vi "ECG AF SPI Input.vi"() -> ()   [LabVIEW 2017]
uses:
  <vilib>/Platform/TimedLoop/XDataNode/wakeup.ctl
  <vilib>/Platform/TimedLoop/XDataNode/XDNodeRunTimeDep.lvlib
  <vilib>/Platform/TimedLoop/XDataNode/nitl_modes.ctl
  <vilib>/Platform/TimedLoop/XDataNode/timing_clust.ctl
  <vilib>/Platform/TimedLoop/XDataNode/XDataNode.xnode
  <vilib>/eio/EIONode/EIONode.xnode
  <vilib>/rvi/eio/common/nirviEmuTemplateMethod_errors.vi
  <vilib>/rvi/Analysis/measure/butterworth/XNode/niFpgaButterworthFilter.xnode
  <vilib>/rvi/Analysis/measure/LMRsmpl/XNode/niFPGA Rational Resampler.xnode
  <vilib>/rvi/LocalResourceManager/LocalResourceManager.xnode
  <vilib>/rvi/DataTransferAndStorage/Container/XNode/niFpgaContainer.xnode
  <vilib>/rvi/FIFO/Fifo_Resource/niFpgaFifoEmulationRefIn.vi
  <vilib>/eio/EIOMethodNode/EIOMethodNode.xnode
  <vilib>/rvi/Analysis/common/codeGenErrors/XNode/niFpgaXNodeCodeGenErrorHandle.vi
  ECG Data.ctl
  Gradient Data.ctl
  All Data.ctl
  IBP Data.ctl
  <vilib>/rvi/DataTransferAndStorage/Container/Common/niFpgaContainerGetUniqueNameForEmu.vi
  <vilib>/rvi/DataTransferAndStorage/Container/Common/niFpgaContainerSetEmuInfo.vi
  <vilib>/rvi/eio/common/nirviEmuReportErrorAndStop.vi
  Trigger Params.ctl
  Channel Enum.ctl
panel:
  in  "IBP Filter":bool
  in  "IBP Offset":fxp<+/-,16,16>
  in  "IBP Scale":fxp<+/-,16,5>=1.0
  in  "Offset":cluster{"X":i16, "Y":i16, "Z":i16}
  in  "Beta IBP":fxp<+/-,32,-16>
  out "IPB1 In":i16
  out "IBP2 In":i16
  out "IPB1 Out":i16
  out "IBP2 Out":i16
  in  "ECG Scale":i16=1 min=1 max=100 step=1
  out "LL Out":i16
  out "LA Out":i16
  out "RA Out":i16
  out "LL In":i16
  out "LA In":i16
  out "RA In":i16
  in  "HPF":bool
  in  "Trigger":T1
  out "IBP Data":T3
  out "ECG Data":T4
  in  "Stop":bool
  in  "Reset":bool
  out "Send":bool
  out "WeightSum":fxp<+/-,33,19> format="%.20g"
  out "BetaProduct":fxp<+/-,32,-1> format="%.33g"
  out "Loop Time":u32
  in  "Filter Size":i16
  out "I In":i16
  out "II In":i16
  out "III In":i16
  out "aVR In":i16
  out "aVL In":i16
  out "aVF In":i16
  out "V1 In":i16
  out "V2 In":i16
  out "V3 In":i16
  out "V4 In":i16
  out "V5 In":i16
  out "V6 In":i16
  out "V4 Out":i16
  out "V5 Out":i16
  out "V6 Out":i16
  out "IBP3":i16
  out "IBP2":i16
  out "IBP1":i16
  in  "Start":bool
  in  "ECG Filter":bool=TRUE
  in  "Beta ECG":fxp<+/-,32,-16>
  out "V3 Out":i16
  out "V2 Out":i16
  out "V1 Out":i16
  out "aVF Out":i16
  out "aVL Out":i16
  out "aVR Out":i16
  out "III Out":i16
  out "II Out":i16
  out "I Out":i16
  out "V6":i16
  out "V5":i16
  out "V4":i16
  out "V3":i16
  out "V2":i16
  out "V1":i16
  out "LL":i16
  out "LA":i16
  out "Actual Loop Rate (Ticks)":u32
  out "Late? Latched":bool
  out "RA":i16
  in  "Loop Rate (Ticks)":u32=4000
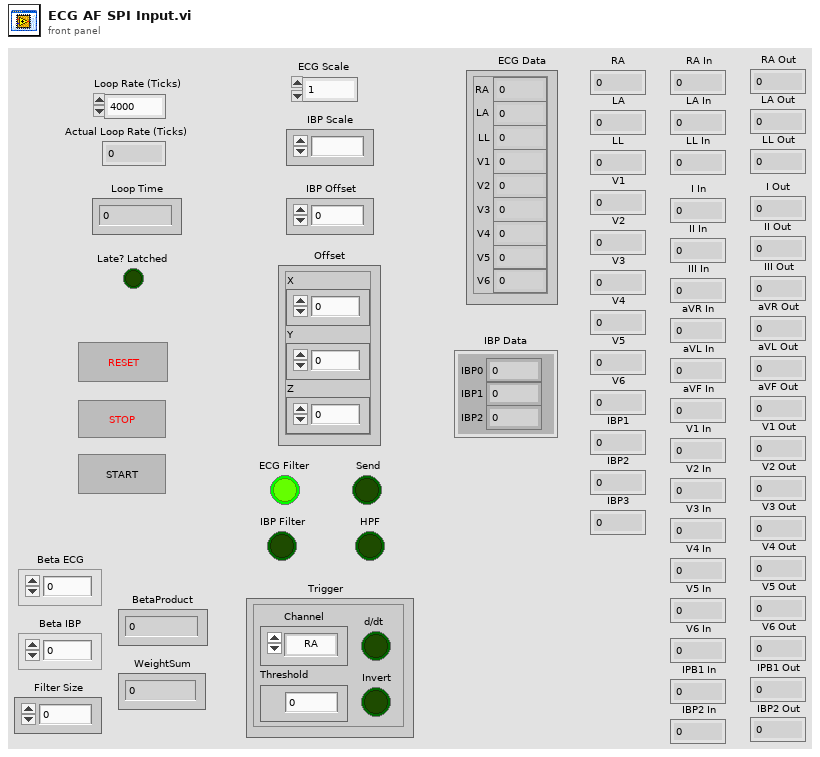
[diagram p1: front panel]
types:
  T1 = typedef "Trigger Params.ctl" = cluster{"Channel":T2, "Threshold":i16, "d/dt":bool, "Invert":bool}
  T2 = typedef "Channel Enum.ctl" = enum16{"RA", "LA", "LL", "V1", "V2", "V3", "V4", "V5", "V6", "I", "II", "III", "aVR", "aVL", "aVF", "Vw", "IBP1", "IBP2"}
  T3 = typedef "IBP Data.ctl" = cluster{"IBP0":fxp<+/-,16,16>, "IBP1":fxp<+/-,16,16>, "IBP2":fxp<+/-,16,16>}
  T4 = typedef "ECG Data.ctl" = cluster{"RA":fxp<+/-,16,16>, "LA":fxp<+/-,16,16>, "LL":fxp<+/-,16,16>, "V1":fxp<+/-,16,16>, "V2":fxp<+/-,16,16>, "V3":fxp<+/-,16,16>, "V4":fxp<+/-,16,16>, "V5":fxp<+/-,16,16>, "V6":fxp<+/-,16,16>}
  T5 = typedef "XDNodeRunTimeDep.lvlib/timing_clust.ctl" = cluster{"Expected End [f-1]":u64, "Actual End [f-1]":u64, "Finished Late? [f-1]":bool, "Expected End [i-1]":u64, "Actual End [i-1]":u64, "Finished Late? [i-1]":bool, "Expected Start [i]":u64, "Actual Start [i]":u64, "Expected Start [f]":u64, "Actual Start [f]":u64, "Source Name":string, "Structure Name":string, "Period":i64, "Deadline":i64, "Offset":i64, "Start":i64, "Priority":i32, "Timeout":i32, "Mode":T6, "Wakeup Reason":T7, "Error":errorcluster, "Source Type":string, "Secondary Source Type":string, "Global End Time":u64, "Global Start Time":u64, "Frame Duration":u64, "Iteration Duration":u64, "Assigned CPU":i32, "I/O Scan Engine Mode":u32}
  T6 = typedef "XDNodeRunTimeDep.lvlib/nitl_modes.ctl" = enum32{"No Change", "Process missed periods, maintain original phase", "Discard missed periods, maintain original phase", "Process missed periods, ignore original phase", "Discard missed periods, ignore original phase"}
  T7 = typedef "XDNodeRunTimeDep.lvlib/wakeup.ctl" = enum32{"Normal", "Aborted", "Asynchronous wakeup", "Timing source error", "Timed loop error", "Timeout"}
  T8 = typedef "Memory Block Channels.ctl" = cluster{"RA":T9, "LA":T9, "LL":T9, "V1":T9, "V2":T9, "V3":T9, "IBP0":T9, "IBP1":T9}
  T9 = typedef "MemoryBlocks.ctl" = cluster{"Taps":refnum<k21>, "Weights":refnum<k21>, "IO Weights":refnum<k21>, "IO Taps":refnum<k21>}
  T10 = cluster{"ECG":cluster{"RA":fxp<+/-,16,16>, "LA":fxp<+/-,16,16>, "LL":fxp<+/-,16,16>, "V1":fxp<+/-,16,16>, "V2":fxp<+/-,16,16>, "V3":fxp<+/-,16,16>, "V4":fxp<+/-,16,16>, "V5":fxp<+/-,16,16>, "V6":fxp<+/-,16,16>}, "Gradients":cluster{"X":fxp<+/-,16,16>, "Y":fxp<+/-,16,16>, "Z":fxp<+/-,16,16>}, "IBP":cluster{"IBP1":fxp<+/-,16,16>, "IBP2":fxp<+/-,16,16>, "IBP3":fxp<+/-,16,16>}}
  T11 = cluster{"BetaProduct":fxp<+/-,32,-1>, "WeightSum":fxp<+/-,33,19>}
  T12 = typedef "ECG Leads.ctl" = cluster{"RA":i16, "LA":i16, "LL":i16, "V1":i16, "V2":i16, "V3":i16, "V4":i16, "V5":i16, "Trigger":i16, "I":i16, "II":i16, "III":i16, "aVR":i16, "aVL":i16, "aVF":i16, "Vw":i16}
  T13 = cluster{"X":fxp<+/-,16,16>, "Y":fxp<+/-,16,16>, "Z":fxp<+/-,16,16>}
  T14 = cluster{"IBP1":fxp<+/-,16,16>, "IBP2":fxp<+/-,16,16>, "IBP3":fxp<+/-,16,16>}
  T15 = typedef "All Data.ctl" = cluster{"ECG":T4, "Gradients":T16, "IBP":T3}
  T16 = typedef "Gradient Data.ctl" = cluster{"X":fxp<+/-,16,16>, "Y":fxp<+/-,16,16>, "Z":fxp<+/-,16,16>}
  T17 = cluster{"IBP0":fxp<+/-,32,21>, "IBP1":fxp<+/-,32,21>, "IBP2":fxp<+/-,32,21>}
  T18 = cluster{"[0]":fxp<+/-,16,16>, "[1]":fxp<+/-,16,16>, "[2]":fxp<+/-,16,16>}
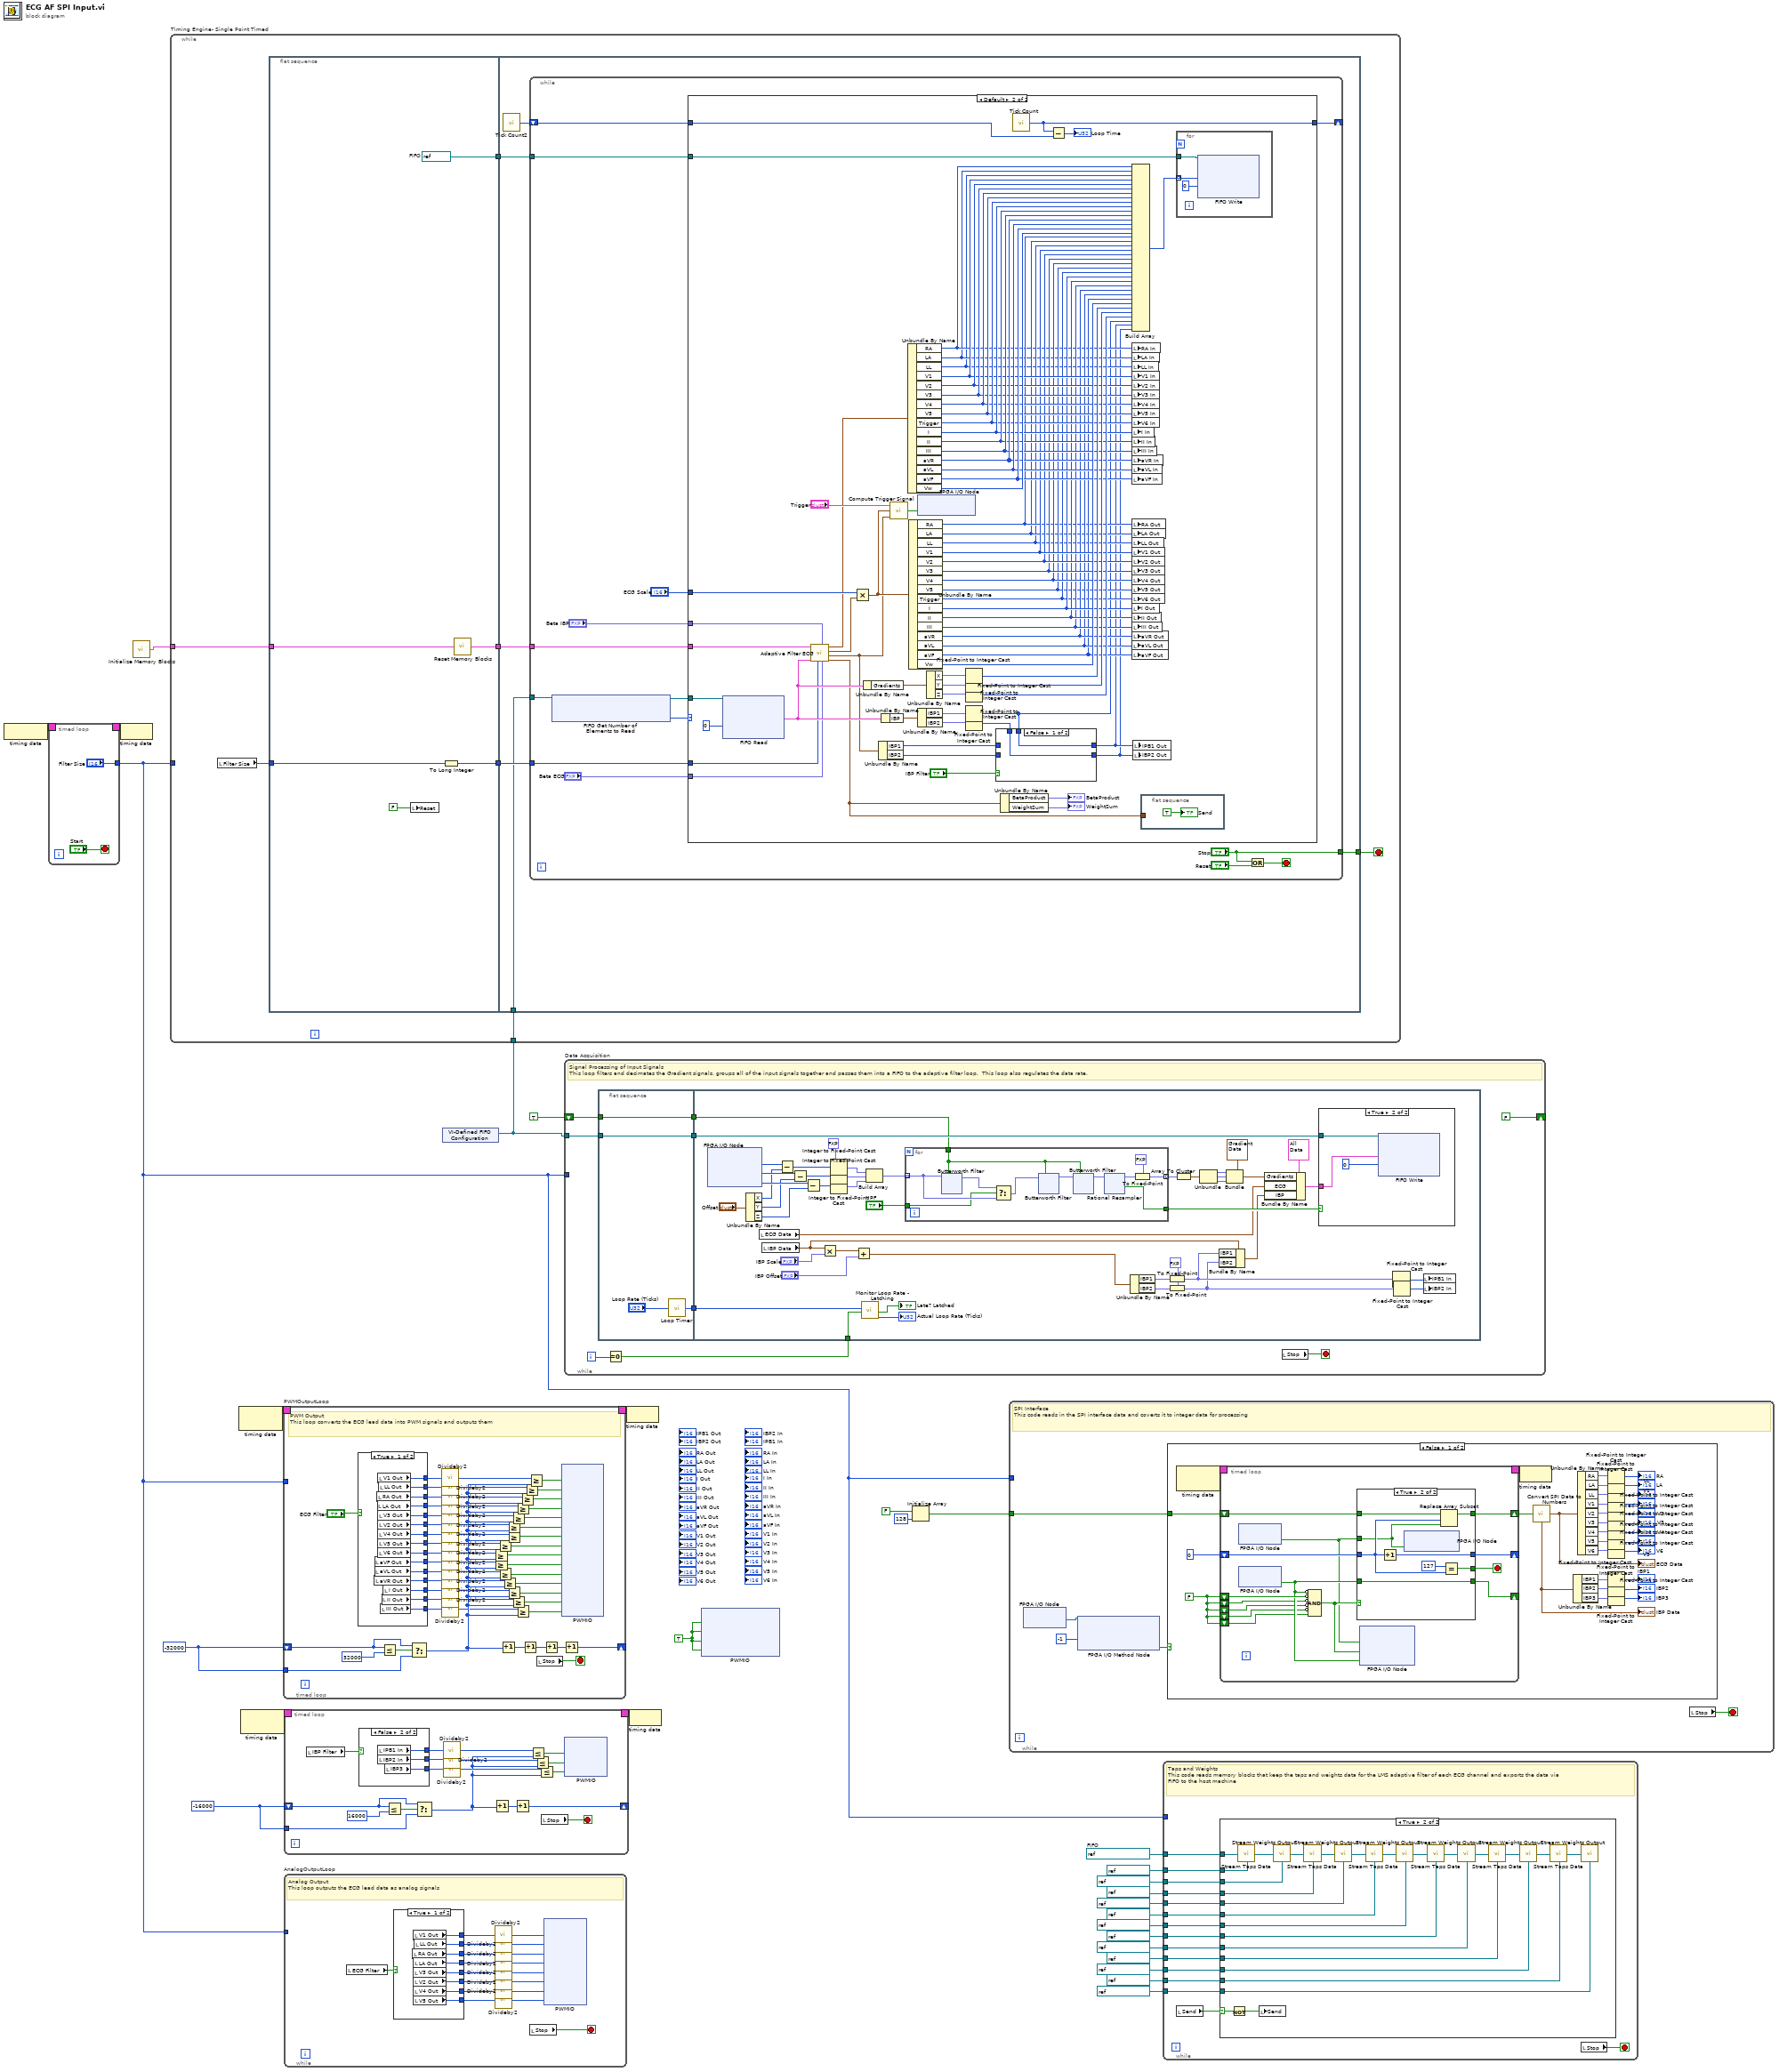
[diagram p0: block diagram]
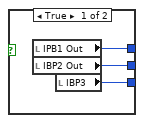
[diagram p2: hidden frame]
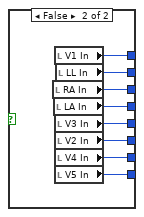
[diagram p5: hidden frame]
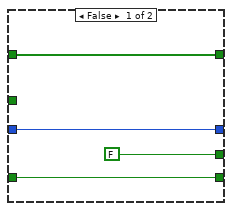
[diagram p6: hidden frame]
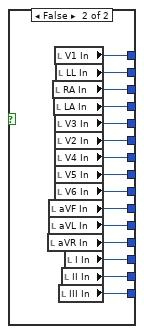
[diagram p8: hidden frame]
diagram:
  w1 = i16 -16000
  w4 = TRUE
  w11 = refnum<k21> "FIFO Filter Specs"  # FIFO
  w27 = i16 -32000
  n1 = node-c288 ("Input Node")() -> (w8:T5)
  n2 = timed-loop "initWait" {
    timing: w8 -> [_]
    timing-out: [_] -> w7
    tunnel: ["Filter Size"] -> w6
    stop <- "Start" stop-if-true
  }
  n3 = node-c288 ("Output Node")(w7) -> ()
  n4 = call "Initialize Memory Blocks.vi"() -> ("Memory"=w10:T8)
  n5 = node-c288 ("Input Node")() -> (w29:T5)  [unwired: 1 in]
  n6 = node-c288() -> (w3:T5)  [unwired: 1 in]
  n7 = timed-loop "PWMOutputLoop" {
    timing: w29 -> [_]
    timing-out: [_] -> w28
    shift-right: [w70] -> _
    shift-left: w27 -> [w87]
    tunnel: w27 -> [w75]
    tunnel: w6 -> [_]
    stop <- w44 stop-if-true
    # "PWM Output\nThis loop converts the ECG lead data into PWM signals and outputs them"
    n8 = case shown="True" "ECG Filter" {
      tunnel: [w104 w119] -> w73
      tunnel: [w103 w118] -> w72
      tunnel: [w102 w117] -> w66
      tunnel: [w101 w116] -> w67
      tunnel: [w100 w115] -> w63
      tunnel: [w99 w114] -> w62
      tunnel: [w98 w113] -> w64
      tunnel: [w97 w112] -> w65
      tunnel: [w96 w111] -> w61
      tunnel: [w95 w110] -> w53
      tunnel: [w94 w109] -> w52
      tunnel: [w93 w108] -> w51
      tunnel: [w92 w107] -> w43
      tunnel: [w91 w106] -> w42
      tunnel: [w90 w105] -> w41
      frame True {
        n9 = local read "aVR Out"() -> (w93:i16)
        n10 = local read "aVF Out"() -> (w95:i16)
        n11 = local read "aVL Out"() -> (w94:i16)
        n12 = local read "RA Out"() -> (w101:i16)
        n13 = local read "LA Out"() -> (w102:i16)
        n14 = local read "V1 Out"() -> (w104:i16)
        n15 = local read "V3 Out"() -> (w97:i16)
        n16 = local read "V2 Out"() -> (w98:i16)
        n17 = local read "V4 Out"() -> (w100:i16)
        n18 = local read "V5 Out"() -> (w99:i16)
        n19 = local read "V6 Out"() -> (w96:i16)
        n20 = local read "LL Out"() -> (w103:i16)
        n21 = local read "III Out"() -> (w90:i16)
        n22 = local read "II Out"() -> (w91:i16)
        n23 = local read "I Out"() -> (w92:i16)
      }
      frame False {
        n24 = local read "aVR In"() -> (w108:i16)
        n25 = local read "aVF In"() -> (w110:i16)
        n26 = local read "aVL In"() -> (w109:i16)
        n27 = local read "RA In"() -> (w116:i16)
        n28 = local read "LA In"() -> (w117:i16)
        n29 = local read "V1 In"() -> (w119:i16)
        n30 = local read "V3 In"() -> (w112:i16)
        n31 = local read "V2 In"() -> (w113:i16)
        n32 = local read "V4 In"() -> (w115:i16)
        n33 = local read "V5 In"() -> (w114:i16)
        n34 = local read "V6 In"() -> (w111:i16)
        n35 = local read "LL In"() -> (w118:i16)
        n36 = local read "III In"() -> (w105:i16)
        n37 = local read "II In"() -> (w106:i16)
        n38 = local read "I In"() -> (w107:i16)
      }
    }
    n39 = Less Or Equal?(x=w87, y=i16 32000 ("Period")) -> (x <= y?=w88:bool)
    n40 = Select(t=w87, s=w88, f=w75) -> (s? t:f=w37:i16)
    n41 = call "Divideby2.vi"("Input"=w73) -> ("Output"=w69:i16)
    n42 = call "Divideby2.vi"("Input"=w72) -> ("Output"=w68:i16)
    n43 = call "Divideby2.vi"("Input"=w67) -> ("Output"=w54:i16)
    n44 = call "Divideby2.vi"("Input"=w66) -> ("Output"=w55:i16)
    n45 = call "Divideby2.vi"("Input"=w65) -> ("Output"=w56:i16)
    n46 = call "Divideby2.vi"("Input"=w64) -> ("Output"=w57:i16)
    n47 = call "Divideby2.vi"("Input"=w63) -> ("Output"=w58:i16)
    n48 = call "Divideby2.vi"("Input"=w62) -> ("Output"=w59:i16)
    n49 = call "Divideby2.vi"("Input"=w61) -> ("Output"=w60:i16)
    n50 = call "Divideby2.vi"("Input"=w53) -> ("Output"=w50:i16)
    n51 = call "Divideby2.vi"("Input"=w52) -> ("Output"=w49:i16)
    n52 = call "Divideby2.vi"("Input"=w51) -> ("Output"=w48:i16)
    n53 = call "Divideby2.vi"("Input"=w43) -> ("Output"=w35:i16)
    n54 = call "Divideby2.vi"("Input"=w42) -> ("Output"=w36:i16)
    n55 = call "Divideby2.vi"("Input"=w41) -> ("Output"=w34:i16)
    n56 = Greater Or Equal?(x=w60, y=w37) -> (x >= y?=w77:bool)
    n57 = Greater Or Equal?(x=w50, y=w37) -> (x >= y?=w47:bool)
    n58 = Greater Or Equal?(x=w59, y=w37) -> (x >= y?=w78:bool)
    n59 = Greater Or Equal?(x=w49, y=w37) -> (x >= y?=w46:bool)
    n60 = Increment(x=w37) -> (x+1=w86:i16)
    n61 = Greater Or Equal?(x=w48, y=w37) -> (x >= y?=w45:bool)
    n62 = Greater Or Equal?(x=w57, y=w37) -> (x >= y?=w80:bool)
    n63 = Greater Or Equal?(x=w58, y=w37) -> (x >= y?=w79:bool)
    n64 = Greater Or Equal?(x=w35, y=w37) -> (x >= y?=w38:bool)
    n65 = Greater Or Equal?(x=w56, y=w37) -> (x >= y?=w81:bool)
    n66 = Greater Or Equal?(x=w36, y=w37) -> (x >= y?=w39:bool)
    n67 = Greater Or Equal?(x=w55, y=w37) -> (x >= y?=w82:bool)
    n68 = Greater Or Equal?(x=w34, y=w37) -> (x >= y?=w40:bool)
    n69 = Greater Or Equal?(x=w54, y=w37) -> (x >= y?=w83:bool)
    n70 = Increment(x=w86) -> (x+1=w74:i16)
    n71 = Greater Or Equal?(x=w68, y=w37) -> (x >= y?=w84:bool)
    n72 = Greater Or Equal?(x=w69, y=w37) -> (x >= y?=w85:bool)
    n73 = local read "Stop"() -> (w44:bool)
    n74 = Increment(x=w74) -> (x+1=w71:i16)
    n75 = xnode ("PWMIO")("V1"=w85, "LL"=w84, "RA"=w83, "LA"=w82, "V3"=w81, "V2"=w80, "V4"=w79, "V5"=w78, "V6"=w77, "aVF"=w47, "aVL"=w46, "aVR"=w45, "I"=w38, "II"=w39, "III"=w40) -> ()  [unwired: 15 in, 15 out]
    n76 = Increment(x=w71) -> (x+1=w70:i16)
  }
  n77 = while "AnalogOutputLoop" {
    tunnel: w6 -> [_]
    stop <- w135 stop-if-true
    # "Analog Output\nThis loop outputs the ECG lead data as analog signals"
    n78 = local read "ECG Filter"() -> (w139:bool)
    n79 = case shown="True" w139 {
      tunnel: [w147 w155] -> w137
      tunnel: [w146 w154] -> w136
      tunnel: [w145 w153] -> w138
      tunnel: [w140 w152] -> w126
      tunnel: [w141 w151] -> w125
      tunnel: [w142 w150] -> w124
      tunnel: [w143 w149] -> w123
      tunnel: [w144 w148] -> w122
      frame True {
        n80 = local read "RA Out"() -> (w142:i16)
        n81 = local read "LA Out"() -> (w141:i16)
        n82 = local read "V1 Out"() -> (w144:i16)
        n83 = local read "V3 Out"() -> (w140:i16)
        n84 = local read "V2 Out"() -> (w145:i16)
        n85 = local read "V4 Out"() -> (w147:i16)
        n86 = local read "V5 Out"() -> (w146:i16)
        n87 = local read "LL Out"() -> (w143:i16)
      }
      frame False {
        n88 = local read "RA In"() -> (w150:i16)
        n89 = local read "LA In"() -> (w151:i16)
        n90 = local read "V1 In"() -> (w148:i16)
        n91 = local read "V3 In"() -> (w152:i16)
        n92 = local read "V2 In"() -> (w153:i16)
        n93 = local read "V4 In"() -> (w155:i16)
        n94 = local read "V5 In"() -> (w154:i16)
        n95 = local read "LL In"() -> (w149:i16)
      }
    }
    n96 = call "Divideby2.vi"("Input"=w122) -> ("Output"=w134:i16)
    n97 = call "Divideby2.vi"("Input"=w123) -> ("Output"=w133:i16)
    n98 = call "Divideby2.vi"("Input"=w124) -> ("Output"=w132:i16)
    n99 = call "Divideby2.vi"("Input"=w125) -> ("Output"=w131:i16)
    n100 = call "Divideby2.vi"("Input"=w126) -> ("Output"=w130:i16)
    n101 = call "Divideby2.vi"("Input"=w138) -> ("Output"=w129:i16)
    n102 = call "Divideby2.vi"("Input"=w137) -> ("Output"=w128:i16)
    n103 = call "Divideby2.vi"("Input"=w136) -> ("Output"=w127:i16)
    n104 = local read "Stop"() -> (w135:bool)
    n105 = xnode ("PWMIO")("ECG0"=w134, "ECG1"=w133, "ECG2"=w132, "ECG3"=w131, "ECG4"=w130, "ECG5"=w129, "ECG6"=w128, "ECG7"=w127) -> ()  [unwired: 8 in, 8 out]
  }
  n106 = timed-loop {
    timing: w3 -> [_]
    timing-out: [_] -> w2
    shift-right: [w156] -> _
    shift-left: w1 -> [w162]
    tunnel: w1 -> [w160]
    stop <- w161 stop-if-true
    n107 = local read "IBP Filter"() -> (w159:bool)
    n108 = case shown="False" w159 {
      tunnel: [w176 w179] -> w170
      tunnel: [w175 w178] -> w169
      tunnel: [w174 w177] -> w168
      frame True {
        n109 = local read "IPB1 Out"() -> (w176:i16)
        n110 = local read "IBP2 Out"() -> (w175:i16)
        n111 = local read "IBP3"() -> (w174:i16)
      }
      frame False {
        n112 = local read "IPB1 In"() -> (w179:i16)
        n113 = local read "IBP2 In"() -> (w178:i16)
        n114 = local read "IBP3"() -> (w177:i16)
      }
    }
    n115 = Less Or Equal?(x=w162, y=i16 16000 ("Period")) -> (x <= y?=w164:bool)
    n116 = Select(t=w162, s=w164, f=w160) -> (s? t:f=w158:i16)
    n117 = call "Divideby2.vi"("Input"=w170) -> ("Output"=w173:i16)
    n118 = call "Divideby2.vi"("Input"=w169) -> ("Output"=w172:i16)
    n119 = call "Divideby2.vi"("Input"=w168) -> ("Output"=w171:i16)
    n120 = Increment(x=w158) -> (x+1=w157:i16)
    n121 = Increment(x=w157) -> (x+1=w156:i16)
    n122 = Less Or Equal?(x=w173, y=w158) -> (x <= y?=w167:bool)
    n123 = Less Or Equal?(x=w172, y=w158) -> (x <= y?=w166:bool)
    n124 = Less Or Equal?(x=w171, y=w158) -> (x <= y?=w165:bool)
    n125 = local read "Stop"() -> (w161:bool)
    n126 = xnode ("PWMIO")("IBP1"=w167, "IBP2"=w166, "IBP3"=w165) -> ()  [unwired: 3 in, 3 out]
  }
  n127 = xnode "VI-Defined FIFO Configuration"() -> ("FIFO Out"=w9:refnum<k21>)
  n128 = while "Timing Engine- Single Point Timed" {
    tunnel: w10 -> [w184]
    tunnel: w9 -> [w183]
    tunnel: w6 -> [_]
    stop <- w185 stop-if-true
    n129 = local read "Filter Size"() -> (w182:i16)
    n130 = flat-sequence "MainSeq" {
      tunnel: [w194] -> w188
      tunnel: [w193] -> w187
      tunnel: [w192] -> w186
      tunnel: w184 -> [w191]
      tunnel: w182 -> [w190]
      tunnel: w188 -> [w200]
      tunnel: w187 -> [w199]
      tunnel: w186 -> [w198]
      tunnel: [w196] -> w185
      tunnel: w183 -> [w195]
      frame #0 {
        w194 = refnum<k21> "FIFO"  # FIFO
        n131 = local write "Reset"(FALSE ("Reset")) -> ()
        n132 = To Long Integer(number=w190) -> (32bit integer=w193:i32)
        n133 = call "Reset Memory Blocks.vi"("Memory Blocks In"=w191) -> ("Memory Blocks Out"=w192:T8)  [unwired: 1 in]
      }
      frame #1 {
        n134 = call "Tick Count2"() -> ("Tick Count(uSec)"=w197:u32)
        n135 = while {
          tunnel: w195 -> [w214]
          tunnel: w200 -> [w210]
          tunnel: w199 -> [w209]
          tunnel: w198 -> [w203]
          shift-right: [w208] -> _
          shift-left: w197 -> [w207]
          tunnel: ["Stop"] -> w196
          stop <- w205 stop-if-true
          n136 = xnode ("FIFO Get Number of Elements to Read")("FIFO In"=w214) -> ("Number of Elements to Read"=w213:u32, "FIFO Out"=w212:refnum<k21>)
          n137 = case shown="Default" w213 {
            tunnel: w212 -> [_ w286]
            tunnel: "Beta ECG" -> [_ w238]
            tunnel: w210 -> [_ w284]
            tunnel: w209 -> [_ w239]
            tunnel: w207 -> [w215 w248]
            tunnel: [w215 w249] -> w208
            tunnel: w203 -> [_ w245]
            tunnel: "ECG Scale" -> [_ w228]
            tunnel: "Beta IBP" -> [_ w225]
            frame 0 {
            }
            frame Default {
              n138 = xnode ("FIFO Read")("Timeout"=0, "FIFO In"=w286) -> ("Element"=w241:T10)  [unwired: 2 out]
              n139 = call "Adaptive Filter ECG.vi"("Beta"=w238, "Beta IBP"=w225, "Filter Length"=w239, "Data in"=w241, "Memory Blocks In"=w245) -> ("Data"=w240:T11, "IBP Out"=w224:cluster{"IBP0":i16, "IBP1":i16}, "Filtered Leads"=w229:T12, "Raw Leads"=w226:T12)  [unwired: 3 in]
              n140 = Multiply(x=w228, y=w229) -> (x*y=w227:T12)
              n141 = Unbundle By Name(w241) -> ("Gradients"=w244:T13)
              n142 = Unbundle By Name(w224) -> ("IBP1"=w220:i16, "IBP2"=w221:i16)
              n143 = Unbundle By Name(w241) -> ("IBP"=w243:T14)
              n144 = call "Compute Trigger Signal.vi"("IBP Out"=w224, "Leads"=w227, "Trigger"="Trigger") -> ("Trigger Out"=w236:bool)
              n145 = Unbundle By Name(w226) -> ("RA"=w232:i16, "LA"=w231:i16, "LL"=w230:i16, "V1"=w263:i16, "V2"=w264:i16, "V3"=w265:i16, "V4"=w266:i16, "V5"=w267:i16, "Trigger"=w268:i16, "I"=w269:i16, "II"=w270:i16, "III"=w271:i16, "aVR"=w272:i16, "aVL"=w273:i16, "aVF"=w274:i16, "Vw"=w279:i16)
              n146 = Unbundle By Name(w227) -> ("RA"=w235:i16, "LA"=w234:i16, "LL"=w233:i16, "V1"=w262:i16, "V2"=w261:i16, "V3"=w260:i16, "V4"=w259:i16, "V5"=w251:i16, "Trigger"=w252:i16, "I"=w258:i16, "II"=w257:i16, "III"=w256:i16, "aVR"=w255:i16, "aVL"=w254:i16, "aVF"=w253:i16, "Vw"=w278:i16)
              n147 = Unbundle By Name(w243) -> ("IBP1"=w242:fxp<+/-,16,16>, "IBP2"=w223:fxp<+/-,16,16>)
              n148 = xnode "FPGA I/O Node"("Trigger Out"=w236) -> ()  [unwired: 1 in, 1 out]
              n149 = Unbundle By Name(w244) -> ("X"=w282:fxp<+/-,16,16>, "Y"=w281:fxp<+/-,16,16>, "Z"=w280:fxp<+/-,16,16>)
              n150 = Fixed-Point to Integer Cast(1:w282) -> (0:w277:i16)
              n151 = Fixed-Point to Integer Cast(1:w281) -> (0:w276:i16)
              n152 = Fixed-Point to Integer Cast(1:w280) -> (0:w275:i16)
              n153 = Fixed-Point to Integer Cast(1:w242) -> (0:w216:i16)
              n154 = Fixed-Point to Integer Cast(1:w223) -> (0:w217:i16)
              n155 = case shown="False" "IBP Filter" {
                tunnel: w221 -> [_ w289]
                tunnel: w220 -> [_ w290]
                tunnel: [w287 w290] -> w219
                tunnel: [w288 w289] -> w218
                tunnel: w217 -> [w288 _]
                tunnel: w216 -> [w287 _]
                frame False {
                }
                frame True {
                }
              }
              n156 = Unbundle By Name(w240) -> ("BetaProduct"=→"BetaProduct":fxp<+/-,32,-1>, "WeightSum"=→"WeightSum":fxp<+/-,33,19>)
              n157 = call "Tick Count"() -> ("Tick Count(uSec)"=w249:u32)
              n158 = Subtract(x=w249, y=w248) -> (x-y=→"Loop Time":u32)
              n159 = Build Array(w232, w231, w230, w263, w264, w265, w266, w267, w268, w269, w270, w271, w272, w273, w274, w279, w235, w234, w233, w262, w261, w260, w259, w251, w252, w258, w257, w256, w255, w254, w253, w278, w277, w276, w275, w216, w219, w218) -> (w283:i16[])
              n160 = local write "RA In"(w232) -> ()
              n161 = local write "LA In"(w231) -> ()
              n162 = local write "LL In"(w230) -> ()
              n163 = local write "V1 In"(w263) -> ()
              n164 = local write "V2 In"(w264) -> ()
              n165 = local write "V3 In"(w265) -> ()
              n166 = local write "V4 In"(w266) -> ()
              n167 = local write "V5 In"(w267) -> ()
              n168 = local write "V6 In"(w268) -> ()
              n169 = local write "I In"(w269) -> ()
              n170 = local write "II In"(w270) -> ()
              n171 = local write "III In"(w271) -> ()
              n172 = local write "aVR In"(w272) -> ()
              n173 = local write "aVL In"(w273) -> ()
              n174 = local write "aVF In"(w274) -> ()
              n175 = local write "RA Out"(w235) -> ()
              n176 = local write "LA Out"(w234) -> ()
              n177 = local write "LL Out"(w233) -> ()
              n178 = local write "V1 Out"(w262) -> ()
              n179 = local write "V2 Out"(w261) -> ()
              n180 = local write "V3 Out"(w260) -> ()
              n181 = local write "V4 Out"(w259) -> ()
              n182 = local write "V5 Out"(w251) -> ()
              n183 = local write "V6 Out"(w252) -> ()
              n184 = local write "I Out"(w258) -> ()
              n185 = local write "II Out"(w257) -> ()
              n186 = local write "III Out"(w256) -> ()
              n187 = local write "aVR Out"(w255) -> ()
              n188 = local write "aVL Out"(w254) -> ()
              n189 = local write "aVF Out"(w253) -> ()
              n190 = local write "IPB1 Out"(w219) -> ()
              n191 = local write "IBP2 Out"(w218) -> ()
              n192 = flat-sequence {
                tunnel: w240 -> [_]
                frame #0 {
                  "Send" <- TRUE ("Send")
                }
              }
              n193 = for {
                tunnel: w284 -> [w294]
                tunnel: w283 -> [w292] mode=indexing
                n194 = xnode ("FIFO Write")("Element"=w292, "Timeout"=0, "FIFO In"=w294) -> ()  [unwired: 2 out]
              }
            }
          }
          n195 = Or(x="Stop", y="Reset") -> (x .or. y?=w205:bool)
        }
      }
    }
  }
  n196 = while "Data Acquisition" {
    tunnel: w9 -> [w302]
    tunnel: w6 -> [_]
    shift-right: [FALSE] -> _
    shift-left: TRUE -> [w297]
    i -> [w300]
    stop <- w298 stop-if-true
    # "Signal Processing of Input Signals\nThis loop filters and decimates the Gradient signals, groups all of the input signals together and passes them into a FIFO to the adaptive filter loop.  This loop also regulates the data rate."
    n197 = flat-sequence "Data Acquisition Sequence" {
      tunnel: ["Loop Rate (Ticks)"] -> w303
      tunnel: w302 -> [w306]
      tunnel: [w306] -> w301
      tunnel: w297 -> [w304]
      tunnel: [w304] -> w296
      tunnel: w303 -> [w350]
      tunnel: w299 -> [w351]
      tunnel: w301 -> [w349]
      tunnel: w296 -> [w328]
      frame #0 {
        n198 = call "Loop Timer"("Count(Ticks)"="Loop Rate (Ticks)") -> ()  [unwired: 1 out]
      }
      frame #1 {
        w310 = fxp<+/-,16,16> 0.0 ("IBP Scale")
        w339 = fxp<+/-,16,16> 0.0 ("fixed-point type")
        n199 = xnode "FPGA I/O Node"() -> ("X Gradient"=w342:i16, "Y Gradient"=w341:i16, "Z Gradient"=w340:i16)  [unwired: 3 in, 3 out]
        n200 = Unbundle By Name("Offset") -> ("X"=w322:i16, "Y"=w320:i16, "Z"=w318:i16)
        n201 = local read "ECG Data"() -> (w329:T4)
        n202 = local read "IBP Data"() -> (w309:T3)
        n203 = Subtract(x=w342, y=w322) -> (x-y=w323:i16)
        n204 = Subtract(x=w341, y=w320) -> (x-y=w321:i16)
        n205 = Subtract(x=w340, y=w318) -> (x-y=w319:i16)
        n206 = Multiply(x=w309, y="IBP Scale") -> (x*y=w316:T17)
        n207 = Integer to Fixed-Point Cast(fixed-point type=w339, integer=w323) -> (fixed-point=w344:fxp<+/-,16,16>)
        n208 = Integer to Fixed-Point Cast(fixed-point type=w339, integer=w321) -> (fixed-point=w345:fxp<+/-,16,16>)
        n209 = Integer to Fixed-Point Cast(fixed-point type=w339, integer=w319) -> (fixed-point=w343:fxp<+/-,16,16>)
        n210 = Add(x=w316, y="IBP Offset") -> (x+y=w308:T17)
        n211 = call "Monitor Loop Rate - Latching.vi"("Reset"=w351, "Count(Ticks)"=w350) -> ("Actual Loop Rate (Ticks)"=→"Actual Loop Rate (Ticks)":u32, "Late? (Latched)"=→"Late? Latched":bool)  [unwired: 7 in, 1 out]
        n212 = Build Array(w344, w345, w343) -> (w346:fxp<+/-,16,16>[])
        n213 = for {
          tunnel: w346 -> [w355] mode=indexing
          tunnel: [w359] -> w338 mode=indexing
          tunnel: [w360] -> w348
          tunnel: w328 -> [w357]
          tunnel: "HPF" -> [w353]
          n214 = xnode "Butterworth Filter"("input data"=w355, "reset"=w357) -> ("output data"=w356:fxp<+/-,16,16>)  [unwired: 1 in, 1 out]
          n215 = Select(t=w356, s=w353, f=w355) -> (s? t:f=w354:fxp<+/-,16,16>)
          n216 = xnode "Butterworth Filter"("input data"=w354, "reset"=w357) -> ("output data"=w363:fxp<+/-,16,16>)  [unwired: 1 in, 1 out]
          n217 = xnode "Butterworth Filter"("input data"=w363, "reset"=w357) -> ("output data"=w362:fxp<+/-,16,16>)  [unwired: 1 in, 1 out]
          n218 = xnode "Rational Resampler"("input data"=w362) -> ("output data"=w361:fxp<+/-,18,16>, "output valid"=w360:bool)  [unwired: 1 out]
          n219 = To Fixed-Point(fixed-point type=fxp<+/-,16,16> 0.0, number=w361) -> (fixed-point=w359:fxp<+/-,16,16>)
        }
        n220 = Unbundle By Name(w308) -> ("IBP1"=w315:fxp<+/-,32,21>, "IBP2"=w314:fxp<+/-,32,21>)
        n221 = To Fixed-Point(fixed-point type=w310, number=w315) -> (fixed-point=w313:fxp<+/-,16,16>)
        n222 = To Fixed-Point(fixed-point type=w310, number=w314) -> (fixed-point=w311:fxp<+/-,16,16>)
        n223 = Array To Cluster(array=w338) -> (cluster=w337:T18)
        n224 = Unbundle(w337) -> ("[0]"=w335:fxp<+/-,16,16>, "[1]"=w334:fxp<+/-,16,16>, "[2]"=w333:fxp<+/-,16,16>)
        n225 = Bundle By Name(cluster=w309, "IBP1"=w313, "IBP2"=w311) -> (w312:T3)
        n226 = Bundle(cluster=T16 {"X"=0.0, "Y"=0.0, "Z"=0.0} ("Gradients"), "X"=w335, "Y"=w334, "Z"=w333) -> (w331:T16)
        n227 = Bundle By Name(cluster=T15 {"ECG"={"RA"=0.0, "LA"=0.0, "LL"=0.0, "V1"=0.0, "V2"=0.0, "V3"=0.0, "V4"=0.0, "V5"=0.0, "V6"=0.0}, "Gradients"={"X"=0.0, "Y"=0.0, "Z"=0.0}, "IBP"={"IBP0"=0.0, "IBP1"=0.0, "IBP2"=0.0}} ("Data"), "Gradients"=w331, "ECG"=w329, "IBP"=w312) -> (w330:T15)
        n228 = case shown="True" w348 {
          tunnel: w349 -> [_ w443]
          tunnel: w330 -> [_ w441]
          frame False {
          }
          frame True {
            n229 = xnode ("FIFO Write")("Element"=w441, "Timeout"=0, "FIFO In"=w443) -> ()  [unwired: 2 out]
          }
        }
        n230 = Fixed-Point to Integer Cast(1:w313) -> (0:w325:i16)
        n231 = Fixed-Point to Integer Cast(1:w311) -> (0:w326:i16)
        n232 = local write "IPB1 In"(w325) -> ()
        n233 = local write "IBP2 In"(w326) -> ()
      }
    }
    n234 = Equal To 0?(x=w300) -> (x = 0?=w299:bool)
    n235 = local read "Stop"() -> (w298:bool)
  }
  n236 = node-c288 ("Output Node")(w28) -> ()
  n237 = node-c288(w2) -> ()
  n238 = xnode ("PWMIO")("Connector0/DIO19"=w4, "Connector0/DIO20"=w4, "Connector0/DIO21"=w4, "Connector0/DIO22"=w4) -> ()  [unwired: 4 in, 4 out]
  n239 = Initialize Array(FALSE, 128 ("dimension size")) -> (w26:bool[])
  n240 = while {
    tunnel: w26 -> [w445]
    tunnel: w6 -> [_]
    stop <- w444 stop-if-true
    # "SPI Interface\nThis code reads in the SPI interface data and coverts it to integer data for processing"
    n241 = xnode "FPGA I/O Node"() -> ("FPGA I/O Out"=w446:refnum<k21>)  [unwired: 1 in, 1 out]
    n242 = xnode "FPGA I/O Method Node"("FPGA I/O In"=w446, "Timeout"=-1) -> ("Timed Out"=w447:bool)  [unwired: 1 out]
    n243 = case shown="False" w447 {
      tunnel: w445 -> [w480 _]
      frame False {
        w476 = FALSE
        n244 = node-c288() -> (w479:T5)  [unwired: 1 in]
        n245 = timed-loop {
          shift-right: [w492] -> w475
          shift-left: w480 -> [w493]
          timing: w479 -> [_]
          timing-out: [_] -> w478
          shift-right: [w488] -> _
          shift-left: w476 -> [w491]
          shift-right: [w489] -> _
          shift-left: u8 0 -> [w490]
          shift-left: w476 -> [w484]
          shift-left: w476 -> [w483]
          shift-left: w476 -> [w482]
          shift-left: w476 -> [w481]
          stop <- w494 stop-if-true
          n246 = xnode "FPGA I/O Node"() -> ("MOSI"=w485:bool)  [unwired: 1 in, 1 out]
          n247 = xnode "FPGA I/O Node"() -> ("SCLK"=w487:bool)  [unwired: 1 in, 1 out]
          n248 = Compound Arithmetic op=AND(invert w487, invert w491, invert w484, invert w483, invert w482, w481) -> (w486:bool)
          n249 = case shown="True" w486 {
            tunnel: [FALSE w505] -> w494
            tunnel: w493 -> [w495 w504]
            tunnel: [w495 w503] -> w492
            tunnel: w490 -> [w498 w502]
            tunnel: [w498 w501] -> w489
            tunnel: w487 -> [w497 w500]
            tunnel: [w497 w500] -> w488
            tunnel: w485 -> [_ w499]
            frame False {
            }
            frame True {
              n250 = Increment(x=w502) -> (x+1=w501:u8)
              n251 = xnode "FPGA I/O Node"("MOSI Data"=w499) -> ()  [unwired: 1 in, 1 out]
              n252 = Replace Array Subset(array=w504, new element=w499, index=w502) -> (w503:bool[])
              n253 = Equal?(x=u8 127, y=w502) -> (x = y?=w505:bool)
            }
          }
          n254 = xnode "FPGA I/O Node"("MOSI Out"=w485, "SCLK Edge"=w486, "SCLK Out"=w487) -> ()  [unwired: 3 in, 3 out]
        }
        n255 = node-c288(w478) -> ()
        n256 = call "Convert SPI Data to Numbers.vi"("Data In"=w475) -> ("IBP Data"=w455:T3, "ECG Data"=w466:T4)
        "ECG Data" <- w466
        "IBP Data" <- w455
        n257 = Unbundle By Name(w455) -> ("IBP1"=w454:fxp<+/-,16,16>, "IBP2"=w452:fxp<+/-,16,16>, "IBP3"=w450:fxp<+/-,16,16>)
        n258 = Unbundle By Name(w466) -> ("RA"=w474:fxp<+/-,16,16>, "LA"=w473:fxp<+/-,16,16>, "LL"=w472:fxp<+/-,16,16>, "V1"=w471:fxp<+/-,16,16>, "V2"=w470:fxp<+/-,16,16>, "V3"=w469:fxp<+/-,16,16>, "V4"=w468:fxp<+/-,16,16>, "V5"=w467:fxp<+/-,16,16>, "V6"=w457:fxp<+/-,16,16>)
        n259 = Fixed-Point to Integer Cast(1:w474) -> (0:→"RA":i16)
        n260 = Fixed-Point to Integer Cast(1:w473) -> (0:→"LA":i16)
        n261 = Fixed-Point to Integer Cast(1:w472) -> (0:→"LL":i16)
        n262 = Fixed-Point to Integer Cast(1:w471) -> (0:→"V1":i16)
        n263 = Fixed-Point to Integer Cast(1:w470) -> (0:→"V2":i16)
        n264 = Fixed-Point to Integer Cast(1:w469) -> (0:→"V3":i16)
        n265 = Fixed-Point to Integer Cast(1:w468) -> (0:→"V4":i16)
        n266 = Fixed-Point to Integer Cast(1:w467) -> (0:→"V5":i16)
        n267 = Fixed-Point to Integer Cast(1:w457) -> (0:→"V6":i16)
        n268 = Fixed-Point to Integer Cast(1:w454) -> (0:→"IBP1":i16)
        n269 = Fixed-Point to Integer Cast(1:w452) -> (0:→"IBP2":i16)
        n270 = Fixed-Point to Integer Cast(1:w450) -> (0:→"IBP3":i16)
      }
      frame True {
      }
    }
    n271 = local read "Stop"() -> (w444:bool)
  }
  n272 = while {
    tunnel: w11 -> [w524]
    tunnel: refnum<k21> "IO Taps 0" ("Memory") -> [w523]
    tunnel: refnum<k21> "IO Weights 0" ("Memory In") -> [w522]
    tunnel: refnum<k21> "IO Taps 1" ("Memory") -> [w521]
    tunnel: refnum<k21> "IO Weights 1" ("Memory In") -> [w520]
    tunnel: refnum<k21> "IO Taps 2" ("Memory") -> [w519]
    tunnel: refnum<k21> "IO Weights 2" ("Memory In") -> [w518]
    tunnel: refnum<k21> "IO Taps 3" ("Memory") -> [w517]
    tunnel: refnum<k21> "IO Weights 3" ("Memory In") -> [w516]
    tunnel: refnum<k21> "IO Taps 4" ("Memory") -> [w515]
    tunnel: refnum<k21> "IO Weights 4" ("Memory In") -> [w514]
    tunnel: refnum<k21> "IO Taps 5" ("Memory") -> [w513]
    tunnel: refnum<k21> "IO Weights 5" ("Memory In") -> [w512]
    tunnel: w6 -> [_]
    stop <- w511 stop-if-true
    # "Taps and Weights\nThis code reads memory blocks that keep the taps and weights data for the LMS adaptive filter of each ECG channel and exports the data via\nFIFO to the host machine"
    n273 = local read "Send"() -> (w525:bool)
    n274 = case shown="True" w525 {
      selector: w525 -> [_ w551]
      tunnel: w524 -> [_ w549]
      tunnel: w523 -> [_ w547]
      tunnel: w522 -> [_ w546]
      tunnel: w521 -> [_ w543]
      tunnel: w520 -> [_ w542]
      tunnel: w519 -> [_ w540]
      tunnel: w518 -> [_ w539]
      tunnel: w517 -> [_ w535]
      tunnel: w516 -> [_ w534]
      tunnel: w515 -> [_ w529]
      tunnel: w514 -> [_ w528]
      tunnel: w513 -> [_ w527]
      tunnel: w512 -> [_ w526]
      frame False {
      }
      frame True {
        n275 = Not(x=w551) -> (.not. x?=w550:bool)
        n276 = call "Stream Taps Data.vi"("FIFO In"=w549, "Memory"=w547) -> ("FIFO out"=w548:refnum<k21>)
        n277 = local write "Send"(w550) -> ()
        n278 = call "Stream Weights Output.vi"("FIFO in"=w548, "Memory In"=w546) -> ("FIFO out"=w544:refnum<k21>)
        n279 = call "Stream Taps Data.vi"("FIFO In"=w544, "Memory"=w543) -> ("FIFO out"=w545:refnum<k21>)
        n280 = call "Stream Weights Output.vi"("FIFO in"=w545, "Memory In"=w542) -> ("FIFO out"=w541:refnum<k21>)
        n281 = call "Stream Taps Data.vi"("FIFO In"=w541, "Memory"=w540) -> ("FIFO out"=w538:refnum<k21>)
        n282 = call "Stream Weights Output.vi"("FIFO in"=w538, "Memory In"=w539) -> ("FIFO out"=w537:refnum<k21>)
        n283 = call "Stream Taps Data.vi"("FIFO In"=w537, "Memory"=w535) -> ("FIFO out"=w536:refnum<k21>)
        n284 = call "Stream Weights Output.vi"("FIFO in"=w536, "Memory In"=w534) -> ("FIFO out"=w530:refnum<k21>)
        n285 = call "Stream Taps Data.vi"("FIFO In"=w530, "Memory"=w529) -> ("FIFO out"=w531:refnum<k21>)
        n286 = call "Stream Weights Output.vi"("FIFO in"=w531, "Memory In"=w528) -> ("FIFO out"=w532:refnum<k21>)
        n287 = call "Stream Taps Data.vi"("FIFO In"=w532, "Memory"=w527) -> ("FIFO out"=w533:refnum<k21>)
        n288 = call "Stream Weights Output.vi"("FIFO in"=w533, "Memory In"=w526) -> ()  [unwired: 1 out]
      }
    }
    n289 = local read "Stop"() -> (w511:bool)
  }
